vi "log creator.vi"() -> ()   [LabVIEW 2012]
uses:
  SubVIs/typedef/Log_User_Data.ctl
  SubVIs/typedef/User Accounts.ctl
panel:
  in  "Log Cluster":T1
  in  "?":bool
  out "CypheredText":string
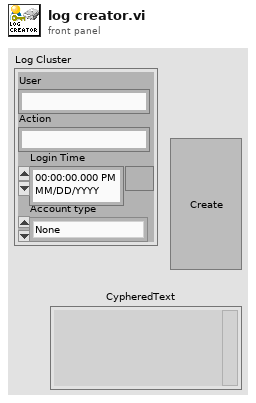
[diagram p1: front panel]
types:
  T1 = typedef "Log_User_Data.ctl" = cluster{"User":string, "Action":string, "Account type":T2, "Login Time ":timestamp}
  T2 = typedef "User Accounts.ctl" = enum16{"None", "User", "Admin"}
  T3 = enum16{"open", "replace", "create", "open or create", "replace or create", "replace or create with confirmation"}
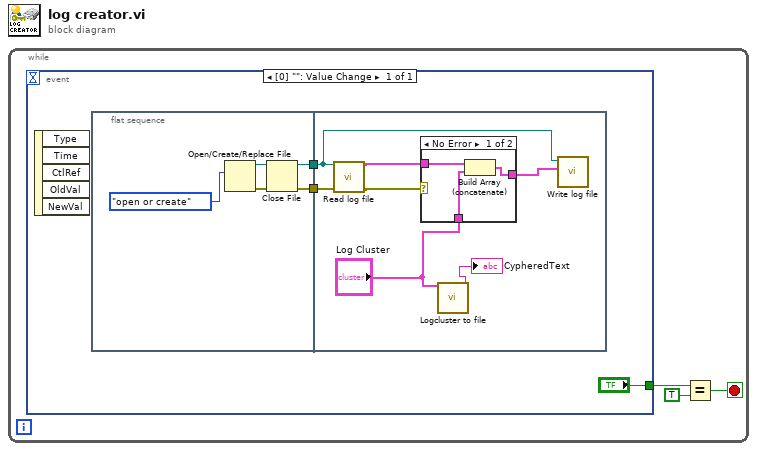
[diagram p0: block diagram]
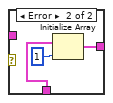
[diagram p2: hidden frame]
diagram:
  n1 = while {
    stop <- w3 stop-if-true
    n2 = event shown="[0] \"\": Value Change" {
      selector: _ -> [_]
      dyn-events: _ -> [_]
      timeout: _ -> [_]
      tunnel: ["?"] -> w1
      event Value Change {
        n3 = event-data() -> ()  [unwired: 1 in, 5 out]
        n4 = flat-sequence {
          tunnel: [w8] -> w5
          tunnel: [w7] -> w4
          tunnel: w5 -> [w15]
          tunnel: w4 -> [w17]
          frame #0 {
            n5 = Open/Create/Replace File(operation (0:open)=T3."open or create") -> (refnum out=w11:refnum<file>, error out=w9:errorcluster)  [unwired: 5 in, 1 out]
            n6 = Close File(refnum=w11, error in=w9) -> (path=w8:path, error out=w7:errorcluster)
          }
          frame #1 {
            n7 = call "Read log file.vi"("file path (use dialog)"=w15, "error in"=w17) -> ("Array"=w18:T1[], "error out"=w16:errorcluster)  [unwired: 12 in]
            n8 = case shown="No Error" w16 {
              tunnel: w18 -> [w21 _]
              tunnel: [w20 w22] -> w14
              tunnel: "Log Cluster" -> [w19 w23]
              frame No Error {
                n9 = Build Array (concatenate)(w21, w19) -> (w20:T1[])
              }
              frame Error {
                n10 = Initialize Array(w23, 1 ("dimension size")) -> (w22:T1[])
              }
            }
            n11 = call "Logcluster to file.vi"("Log Cluster"="Log Cluster") -> ("CypheredText"=→"CypheredText":string)  [unwired: 13 in, 1 out]
            n12 = call "Write log file.vi"("UDcluster Array in"=w14, "file path (use dialog)"=w15) -> ()  [unwired: 8 in, 2 out]
          }
        }
      }
    }
    n13 = Equal?(x=w1, y=TRUE) -> (x = y?=w3:bool)
  }
